vi "Get Energy.vi"(10 "Beam":refnum<class "Beam.lvclass">, 11 "Maze in":refnum<class "Maze.lvclass">) -> (2 "Numeric":i32, 3 "Maze Out":refnum<class "Maze.lvclass">)   [LabVIEW 2021, in "Maze.lvclass"]
uses:
  Maze.lvclass
  Beam/Beam.lvclass
  Maze.lvclass/Maze.ctl
  Beam/Beam.lvclass/Beam.ctl
  Beam/Read Row.vi
  Beam/Read Col.vi
panel:
  out "Array":bool[][](array[boolean])
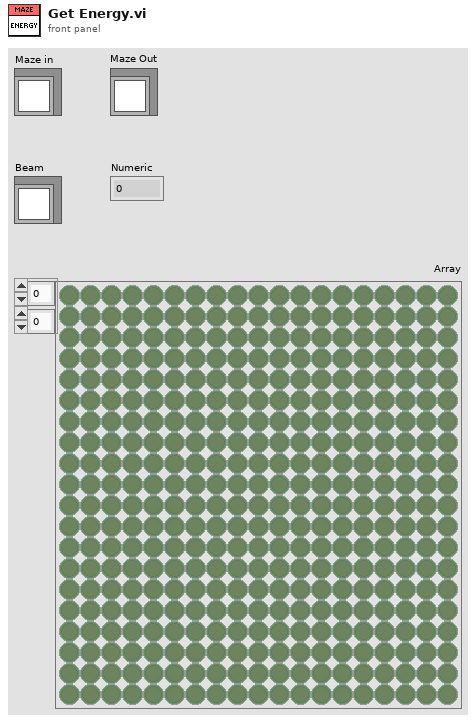
[diagram p1: front panel]
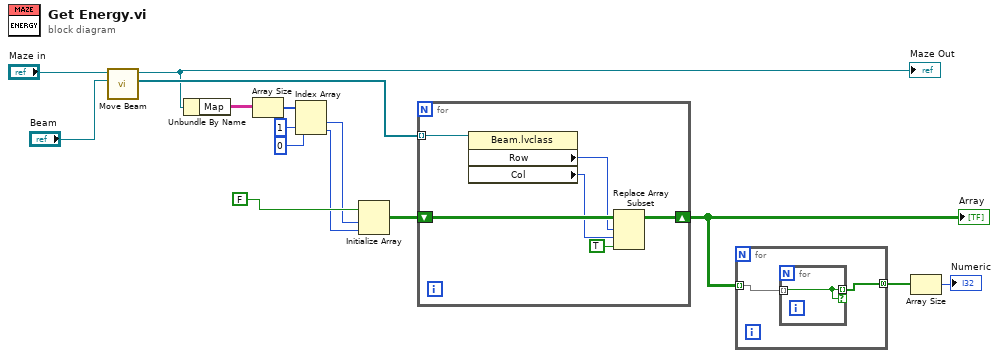
[diagram p0: block diagram]
diagram:
  n1 = call "Move Beam.vi"("Beam"="Beam", "Maze In"="Maze in") -> ("Beams"=w11:refnum<class "Beam.lvclass">[], "Maze Out"=w3:refnum<class "Maze.lvclass">)  [unwired: 8 in]
  "Maze Out" <- w3
  n2 = Unbundle By Name(w3) -> ("Map"=w7:string[][])
  n3 = Array Size(array=w7) -> (size(s)=w6:i32[])
  n4 = Index Array(array=w6, index #1=1 ("index"), index #2=0 ("index")) -> (element #1=w5:i32, element #2=w4:i32)
  n5 = Initialize Array(FALSE, w5, w4) -> (w13:bool[][])
  n6 = for {
    tunnel: w11 -> [w21] mode=indexing
    shift-right: [w16] -> w9
    shift-left: w13 -> [w20]
    n7 = property class="Beam.lvclass"(reference=w21) -> ("Row"=w19:i32, "Col"=w18:i32)  [unwired: 1 in, 2 out]
    n8 = Replace Array Subset(array=w20, new element=TRUE ("new element/subarray"), index (row)=w19, index (col)=w18) -> (w16:bool[][])
  }
  "Array" <- w9
  n9 = for {
    tunnel: w9 -> [w23] mode=indexing
    tunnel: [w22] -> w14 mode=concatenating
    n10 = for {
      tunnel: w23 -> [w24] mode=indexing
      tunnel: [w24] -> w22 mode=indexing if=w24
    }
  }
  n11 = Array Size(array=w14) -> (size(s)=→"Numeric":i32)
